vi "Check Name.vi"(11 "shared memory name in":string) -> (3 "shared memory name out":string)   [LabVIEW 2013, in "Shared Memory.lvlib" / "Shared Memory.lvclass"]
doc: "Checks the provided string name for shm_open() and ensure that there is a leading '/' character to comply with the formatting expected by shm_open()."
uses:
  Shared Memory.lvclass
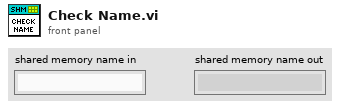
[diagram p1: front panel]
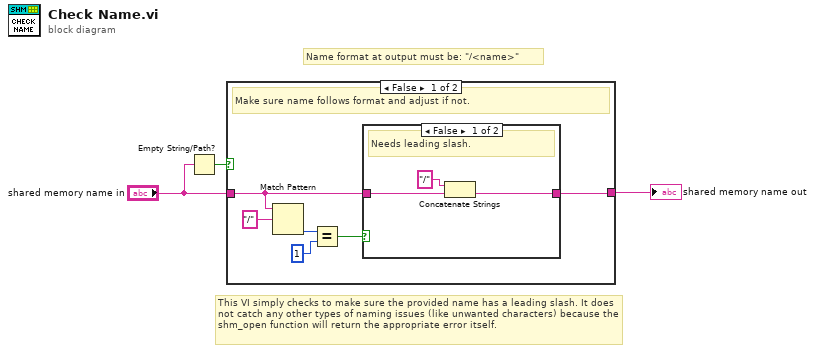
[diagram p0: block diagram]
diagram:
  # "This VI simply checks to make sure the provided name has a leading slash. It does not catch any other types of naming issues (like unwanted characters) because the shm_open function will return the appropriate error itself."
  # "Name format at output must be: \"/<name>\""
  n1 = Empty String/Path?(string/path="shared memory name in") -> (empty?=w1:bool)
  n2 = case shown="False" w1 {
    tunnel: [w4 w14] -> w3
    tunnel: "shared memory name in" -> [w6 w14]
    frame False {
      # "Make sure name follows format and adjust if not."
      n3 = Match Pattern(string=w6, regular expression="/") -> (offset past match=w7:i32)  [unwired: 1 in, 3 out]
      n4 = Equal?(x=w7, y=1) -> (x = y?=w5:bool)
      n5 = case shown="False" w5 {
        tunnel: w6 -> [w12 w13]
        tunnel: [w11 w13] -> w4
        frame False {
          # "Needs leading slash."
          n6 = Concatenate Strings("/", w12) -> (w11:string)
        }
        frame True {
          # "Has leading slash. Passthru."
        }
      }
    }
    frame True {
      # "Empty string. Shm_open will generate error."
    }
  }
  "shared memory name out" <- w3
